vi "Cannon Global Data.vi"() -> ()   [LabVIEW 2012]
panel:
  in  "Cannon Global Data":T1
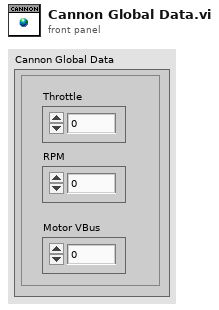
[diagram p1: front panel]
types:
  T1 = cluster{"Throttle":dbl, "RPM":dbl, "Motor VBus":dbl}
diagram:
